vi "GE 5565PIORC.DMA.Block.Write (Pointer).vi"(7 "bytes to move":u32, 8 "error in (no error)":errorcluster, 9 "src pointer":u64, 10 "Block Descriptor in":T1 {"descriptor params"."data ptr (lower)" format="%.0x"; "descriptor params"."data ptr (upper)" format="%.0x"; "descriptor params"."data size" format="%.0x"; "descriptor params"."next descriptor ptr" format="%.0x"; "descriptor size" format="%08x"; "descriptor ptr (RFM)" format="%08x"; "descriptor ptr (VISA)" format="%08x"}, 11 "GE 5565PIORC in":refnum<class "GE 5565PIORC.lvclass">) -> (0 "error out":errorcluster, 1 "src pointer out":u64, 2 "Block Descriptor out":T1 {"descriptor params"."data ptr (lower)" format="%.0x"; "descriptor params"."data ptr (upper)" format="%.0x"; "descriptor params"."data size" format="%.0x"; "descriptor params"."next descriptor ptr" format="%.0x"; "descriptor size" format="%08x"; "descriptor ptr (RFM)" format="%08x"; "descriptor ptr (VISA)" format="%08x"}, 3 "GE 5565PIORC out":refnum<class "GE 5565PIORC.lvclass">)   [LabVIEW 2016, in "GE 5565PIORC.lvclass"]
doc: "Moves data from <B>src pointer</B> to the specified <B>Block Descriptor</B>. The number of bytes transferred will be either the requested <B>bytes to move</B> or the size of the block specified by <B>Block Descriptor</B>, whichever is smaller."
uses:
  GE 5565PIORC.lvclass
  Typedefs/GE 5565PIORC.Typedef.DMA Block Descriptor.ctl
  Typedefs/GE 5565PIORC.Typedef.DMA Block Descriptor Params.ctl
  GE 5565PIORC.lvclass/GE 5565PIORC.ctl
  <vilib>/Instr/_visa.llb/VISA Register Access Address Space.ctl
  GE 5565PIORC.DMA.Block.VISA Return Handler.vi
  <vilib>/Utility/error.llb/Error Cluster From Error Code.vi
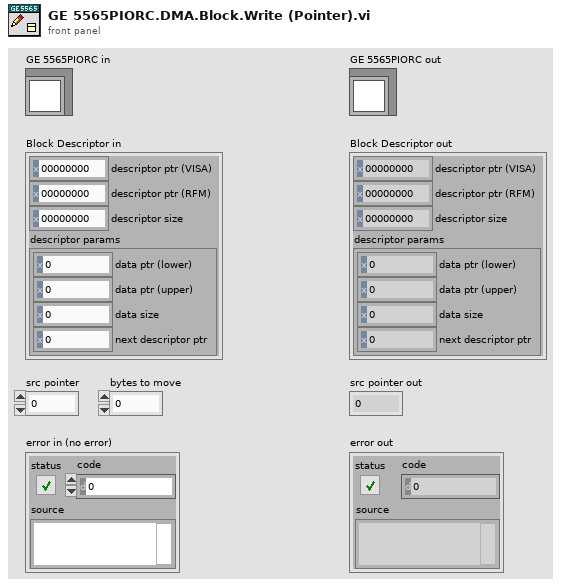
[diagram p1: front panel]
types:
  T1 = typedef "GE 5565PIORC.lvclass/GE 5565PIORC.Typedef.DMA Block Descriptor.ctl" = cluster{"descriptor ptr (VISA)":u32, "descriptor ptr (RFM)":u32, "descriptor size":u32, "descriptor params":T2}
  T2 = typedef "GE 5565PIORC.lvclass/GE 5565PIORC.Typedef.DMA Block Descriptor Params.ctl" = cluster{"data ptr (lower)":u32, "data ptr (upper)":u32, "data size":u32, "next descriptor ptr":u32}
  T3 = typedef "VISA Register Access Address Space.ctl" = u16
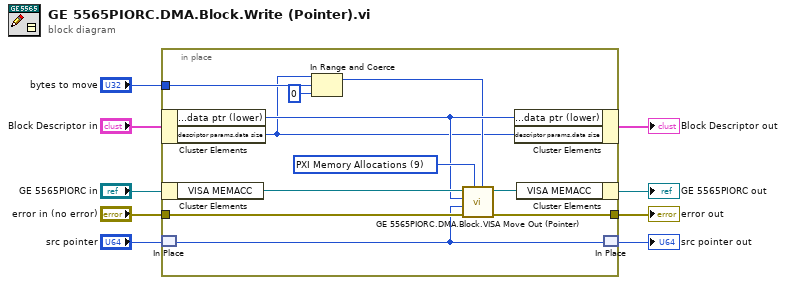
[diagram p0: block diagram]
diagram:
  n1 = in-place {
    in-place-border: "error in (no error)" -> [w20]
    in-place-border: [w19] -> w8
    in-place-border: "bytes to move" -> [w14]
    w16 = T3 9 items=["VXI/VME A16"=1, "VXI/VME A24"=2, "VXI/VME A32"=3, "VXI/VME A64"=4, "PXI Memory Allocations"=9, "PXI Configuration"=10, "PXI BAR0"=11, "PXI BAR1"=12, "PXI BAR2"=13, "PXI BAR3"=14, "PXI BAR4"=15, "PXI BAR5"=16] ("address space")
    n2 = in-place-cluster #1("Block Descriptor in") -> ("descriptor params.data ptr (lower)"=w12:u32, "descriptor params.data size"=w10:u32)
    n3 = in-place-cluster #2("GE 5565PIORC in") -> ("VISA MEMACC"=w18:refnum<visa-resource-name>)
    n4 = in-place-match #3("src pointer") -> (w15:u64)
    n5 = In Range and Coerce(upper limit=w10, x=w14, lower limit=u32 0) -> (coerced(x)=w11:u32)  [unwired: 1 out]
    n6 = call "GE 5565PIORC.DMA.Block.VISA Move Out (Pointer).vi"("bytes to move"=w11, "address space"=w16, "error in (no error)"=w20, "src pointer"=w15, "offset (0)"=w12, "VISA resource name"=w18) -> ("error out"=w19:errorcluster, "VISA resource name out"=w17:refnum<visa-resource-name>)  [unwired: 4 in]
    n7 = in-place-cluster #1("descriptor params.data ptr (lower)"=w12, "descriptor params.data size"=w10) -> (→"Block Descriptor out":T1)
    n8 = in-place-cluster #2("VISA MEMACC"=w17) -> (→"GE 5565PIORC out":refnum<class "GE 5565PIORC.lvclass">)
    n9 = in-place-match #3(w15) -> (→"src pointer out":u64)
  }
  "error out" <- w8
